vi "Motor to TDMS.vi"(5 "Target Torque":i16(knob) scale=-1000.0..1000.0, 7 "Motor Status":T1, 8 "error in (no error)":errorcluster, 9 "Timestamp":u32, 10 "group name in (Untitled)":string, 11 "tdms file":refnum<k34>) -> (0 "error out":errorcluster, 2 "group name out":string, 3 "tdms file out":refnum<k34>)   [LabVIEW 2016]
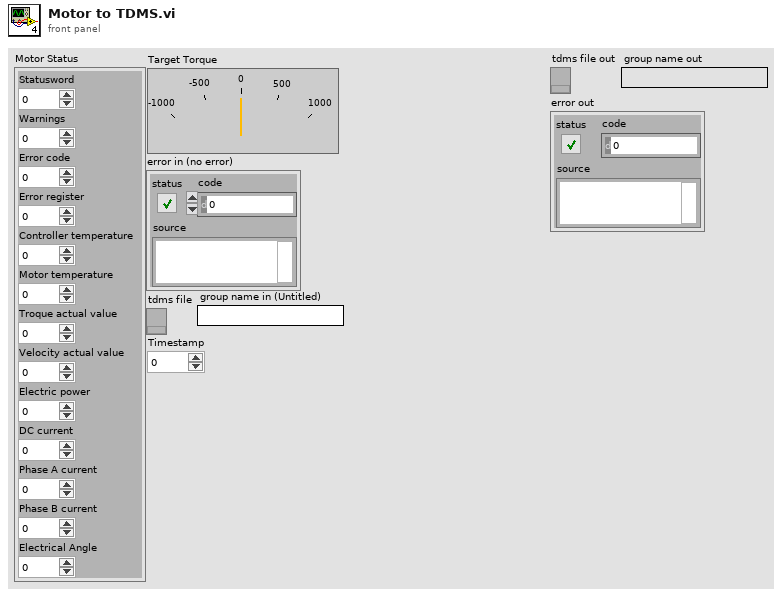
[diagram p1: front panel]
types:
  T1 = cluster{"Statusword":u16, "Warnings":u16, "Error code":u16, "Error register":u8, "Controller temperature":u8, "Motor temperature":u8, "Troque actual value":i16, "Velocity actual value":i32, "Electric power":u32, "DC current":u32, "Phase A current":u16, "Phase B current":u16, "Electrical Angle":u16}
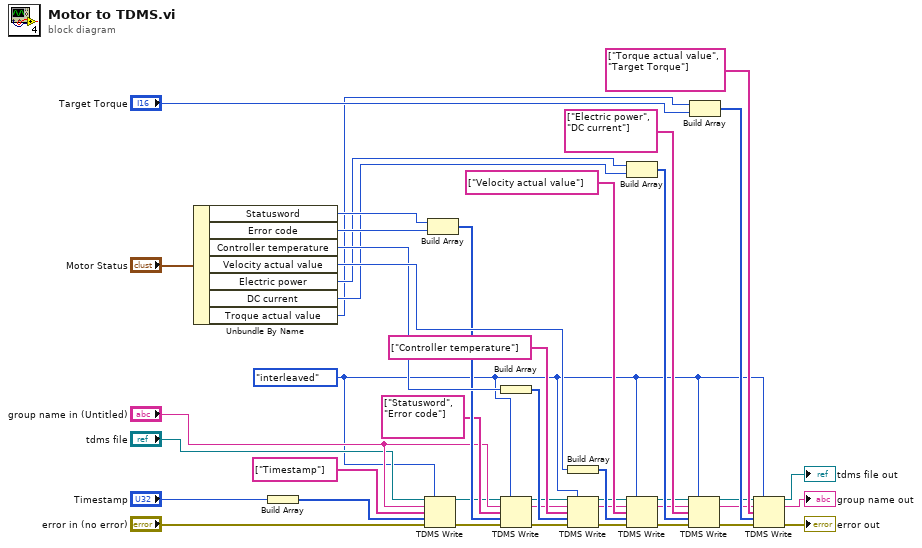
[diagram p0: block diagram]
diagram:
  w1 = enum16{"decimated", "interleaved"}."interleaved" ("data layout (0:decimated)")
  n1 = Unbundle By Name("Motor Status") -> ("Statusword"=w43:u16, "Error code"=w41:u16, "Controller temperature"=w40:u8, "Velocity actual value"=w42:i32, "Electric power"=w39:u32, "DC current"=w36:u32, "Troque actual value"=w35:i16)
  n2 = Build Array("Timestamp") -> (w6:u32[])
  n3 = TDMS Write(0:"tdms file", 1:w1, 5:"group name in (Untitled)", 7:string[] ["Timestamp"] ("channel name(s) in (Untitled)"), 9:w6, 11:"error in (no error)") -> (4:w2:refnum<k34>, 15:w4:errorcluster)  [unwired: 2 out]
  n4 = Build Array(w43, w41) -> (w34:u16[])
  n5 = Build Array(w40) -> (w33:u8[])
  n6 = TDMS Write(0:w2, 1:w1, 5:"group name in (Untitled)", 7:string[] ["Statusword", "Error code"] ("channel name(s) in (Untitled)"), 9:w34, 11:w4) -> (4:w16:refnum<k34>, 6:w20:string, 15:w30:errorcluster)  [unwired: 1 out]
  n7 = Build Array(w42) -> (w32:i32[])
  n8 = TDMS Write(0:w16, 1:w1, 5:w20, 7:string[] ["Controller temperature"] ("channel name(s) in (Untitled)"), 9:w33, 11:w30) -> (4:w15:refnum<k34>, 6:w19:string, 15:w29:errorcluster)  [unwired: 1 out]
  n9 = Build Array(w39, w36) -> (w31:u32[])
  n10 = TDMS Write(0:w15, 1:w1, 5:w19, 7:string[] ["Velocity actual value"] ("channel name(s) in (Untitled)"), 9:w32, 11:w29) -> (4:w14:refnum<k34>, 6:w18:string, 15:w28:errorcluster)  [unwired: 1 out]
  n11 = TDMS Write(0:w14, 1:w1, 5:w18, 7:string[] ["Electric power", "DC current"] ("channel name(s) in (Untitled)"), 9:w31, 11:w28) -> (4:w13:refnum<k34>, 6:w17:string, 15:w26:errorcluster)  [unwired: 1 out]
  n12 = Build Array(w35, "Target Torque") -> (w27:i16[])
  n13 = TDMS Write(0:w13, 1:w1, 5:w17, 7:string[] ["Torque actual value", "Target Torque"] ("channel name(s) in (Untitled)"), 9:w27, 11:w26) -> (4:→"tdms file out":refnum<k34>, 6:→"group name out":string, 15:→"error out":errorcluster)  [unwired: 1 out]
